vi "MS SQL_InRFID_STN30B.vi"(6 "RFID":string, 7 "OP30B_006_CIRCLIP_MEAS":T1, 8 "error in (no error)":errorcluster, 11 "Ref in":T2={"MS SQL Connection"=refnum, "UDL File"=path "", "Time"="", "DCODE"="", "WIP+1"=0, "MC No?"=0, "POKAYOKE?"=FALSE, "Expected Result"="", "Result [Status]"="", "Clock"=0.0, "RFID"="", "WIP Queue"=refnum, "TS Parameter"={"ProfitCenterCode"="", "LineCode"="", "WorkOrderNumber"="", "Model"="", "Model_with_Prefix"="", "VendorCode"="", "SetParameterDateCode"="", "PokaYoke"=0, "Target"=1, "Live_DateCode"="", "CustomerPartNumber"="", "Hand"="", "Ent_Stamp"=timestamp(0 s since 1904-01-01), "STS_CD"=0.0}, "Data_Queue"=[], "RFID Serial No."=""} {"TS Parameter"."Target" min=1 max=100000; "TS Parameter"."PokaYoke" min=0 max=1}) -> (0 "error out":errorcluster, 1 "Message":picture, 3 "Ref Out":T2={"MS SQL Connection"=refnum, "UDL File"=path "", "Time"="", "DCODE"="", "WIP+1"=0, "MC No?"=0, "POKAYOKE?"=FALSE, "Expected Result"="", "Result [Status]"="", "Clock"=0.0, "RFID"="", "WIP Queue"=refnum, "TS Parameter"={"ProfitCenterCode"="", "LineCode"="", "WorkOrderNumber"="", "Model"="", "Model_with_Prefix"="", "VendorCode"="", "SetParameterDateCode"="", "PokaYoke"=0, "Target"=1, "Live_DateCode"="", "CustomerPartNumber"="", "Hand"="", "Ent_Stamp"=timestamp(0 s since 1904-01-01), "STS_CD"=0.0}, "Data_Queue"=[], "RFID Serial No."=""} {"TS Parameter"."Target" min=1 max=100000; "TS Parameter"."PokaYoke" min=0 max=1})   [LabVIEW 2020]
uses:
  Controls/TD SQL.ctl
  <vilib>/addons/database/Connection.llb/Conn ObjectReference.ctl
  Controls/WIP_State.ctl
  Controls/TS_Parameter.ctl
  Controls/OP30B_DataCluster.ctl
  <vilib>/addons/database/NI_Database_API.lvlib
panel:
  out "OP30B VISION STATUS":i32
  out "resulting string":string
  # "OP60"
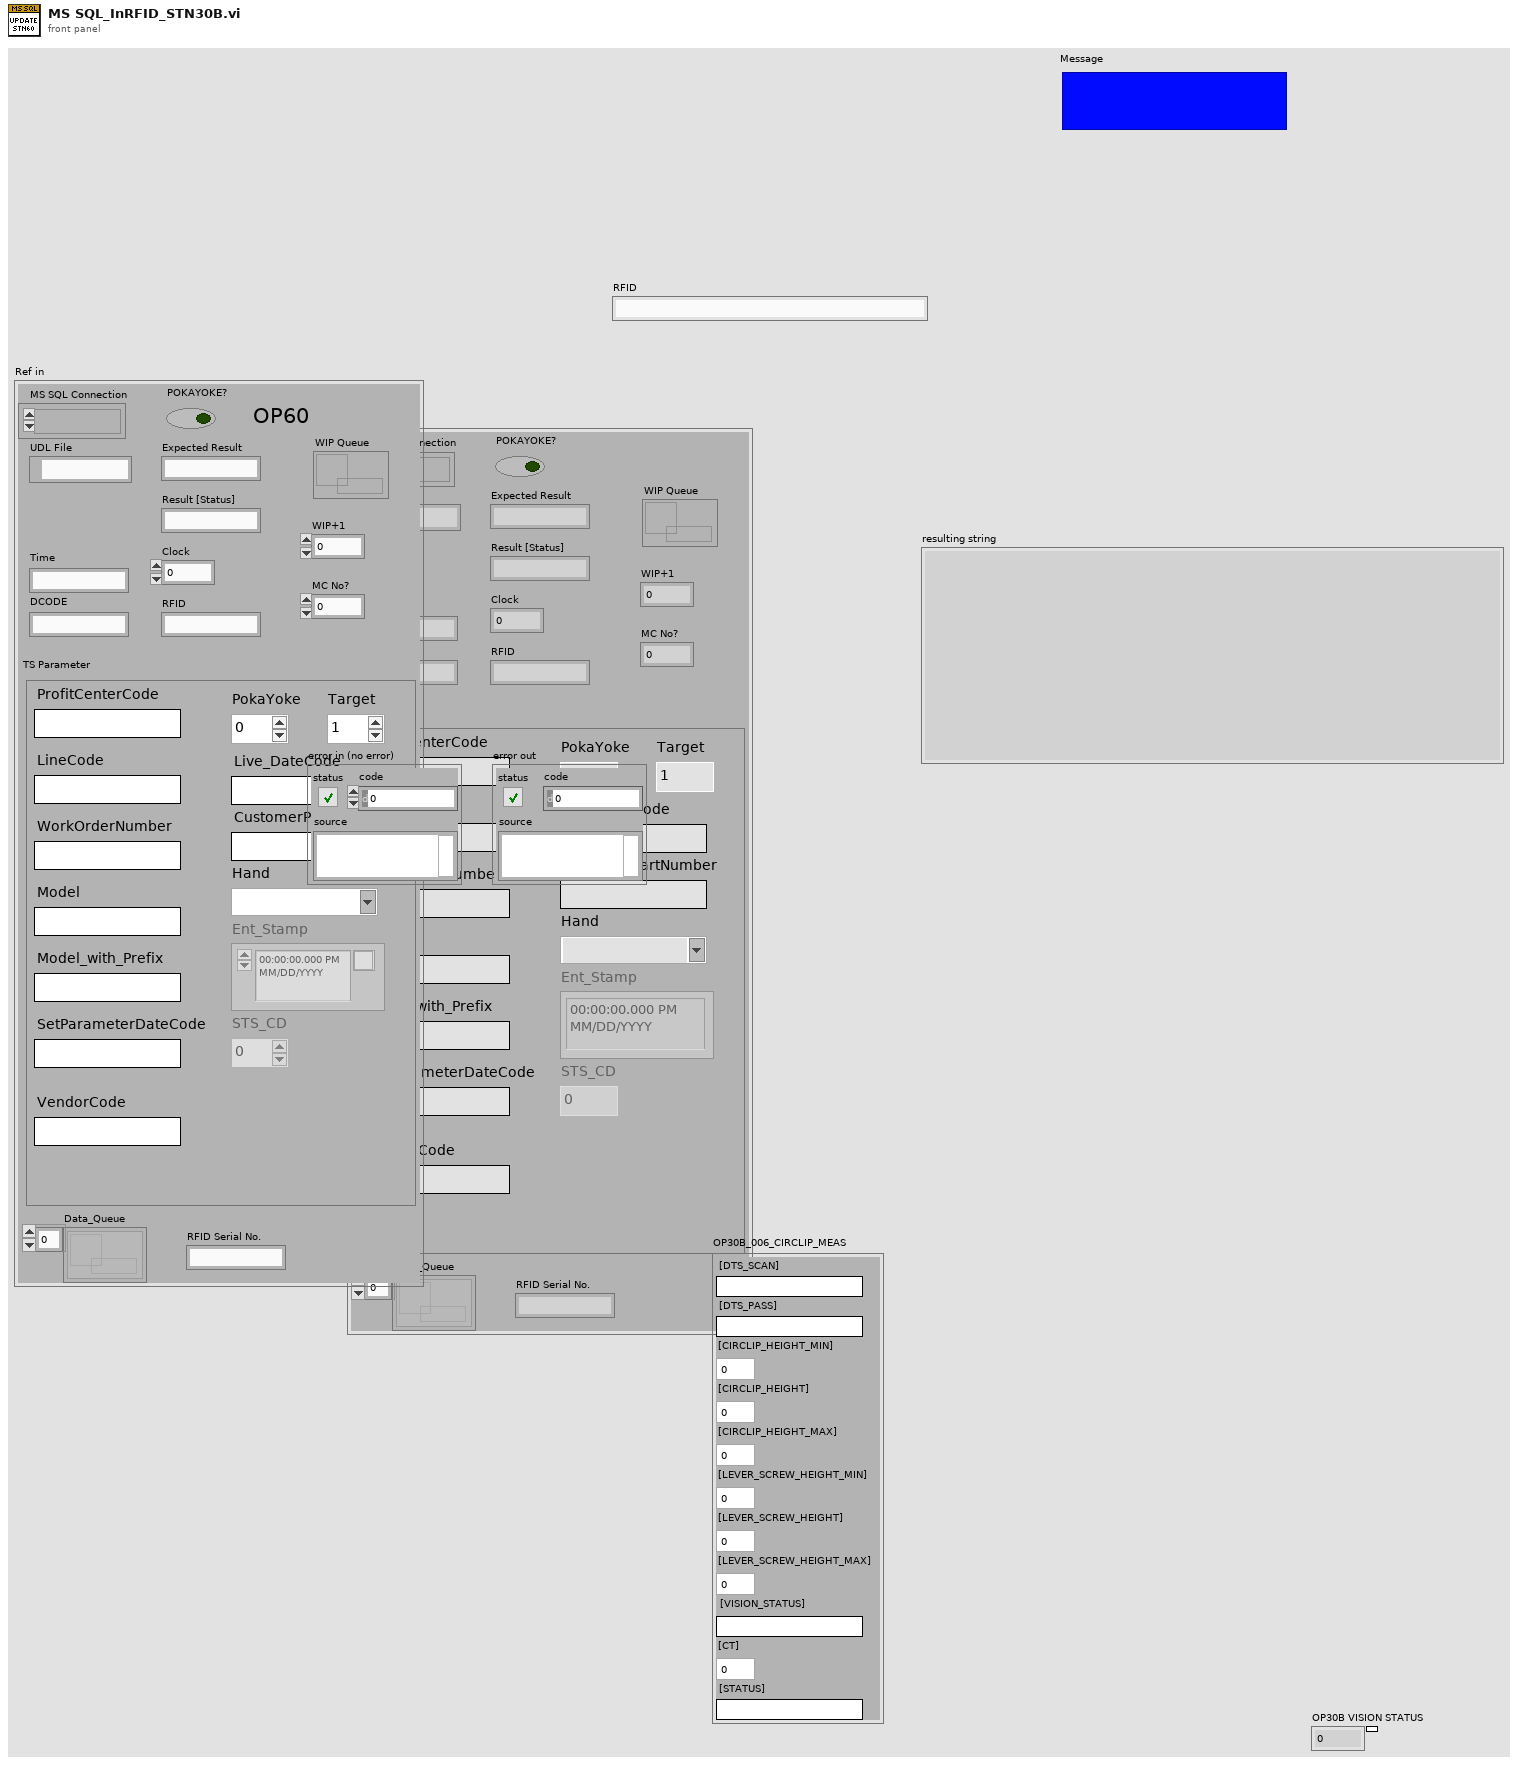
[diagram p1: front panel]
types:
  T1 = typedef "OP30B_DataCluster.ctl" = cluster{"[DTS_SCAN]":string, "[DTS_PASS]":string, "[CIRCLIP_HEIGHT_MIN]":dbl, "[CIRCLIP_HEIGHT]":dbl, "[CIRCLIP_HEIGHT_MAX]":dbl, "[LEVER_SCREW_HEIGHT_MIN]":dbl, "[LEVER_SCREW_HEIGHT]":dbl, "[LEVER_SCREW_HEIGHT_MAX]":dbl, "[VISION_STATUS]":string, "[CT]":dbl, "[STATUS]":string}
  T2 = typedef "TD SQL.ctl" = cluster{"MS SQL Connection":T3, "UDL File":path, "Time":string, "DCODE":string, "WIP+1":i64, "MC No?":i32, "POKAYOKE?":bool, "Expected Result":string, "Result [Status]":string, "Clock":dbl, "RFID":string, "WIP Queue":refnum<queue>, "TS Parameter":T4, "Data_Queue":refnum<queue>[], "RFID Serial No.":string}
  T3 = typedef "NI_Database_API.lvlib/Conn ObjectReference.ctl" = refnum<k1>
  T4 = typedef "TS_Parameter.ctl" = cluster{"ProfitCenterCode":string, "LineCode":string, "WorkOrderNumber":string, "Model":string, "Model_with_Prefix":string, "VendorCode":string, "SetParameterDateCode":string, "PokaYoke":i32, "Target":i32, "Live_DateCode":string, "CustomerPartNumber":string, "Hand":string, "Ent_Stamp":timestamp, "STS_CD":dbl}
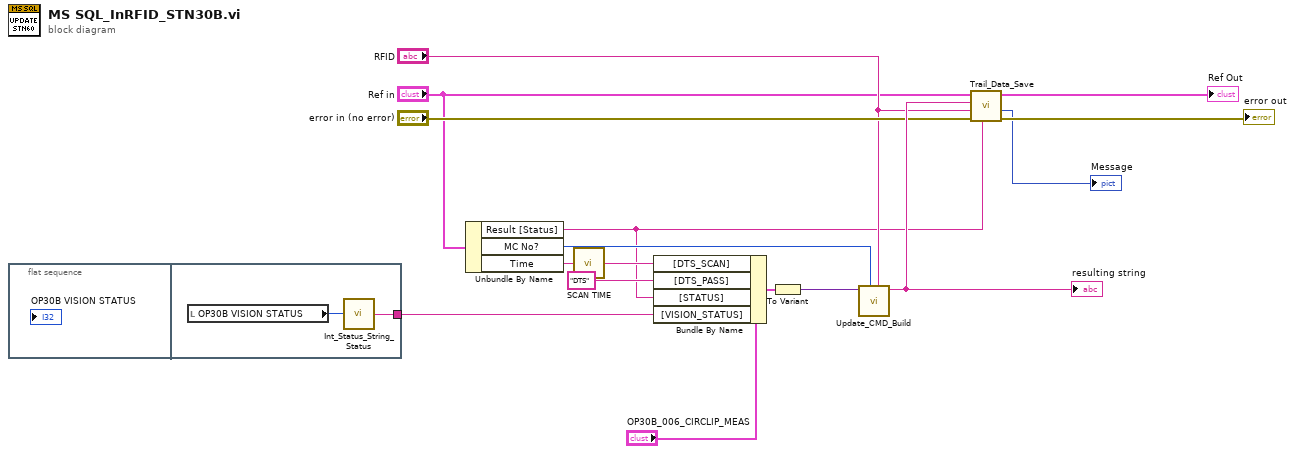
[diagram p0: block diagram]
diagram:
  n1 = flat-sequence {
    tunnel: [w17] -> w3
    frame #0 {
    }
    frame #1 {
      n2 = local read "OP30B VISION STATUS"() -> (w18:i32)
      n3 = call "Int_Status_String_Status.vi"("[STATUS]"=w18) -> ("STATUS"=w17:string)
    }
  }
  n4 = Unbundle By Name("Ref in") -> ("Result [Status]"=w1:string, "MC No?"=w2:i32, "Time"=w6:string)
  n5 = call "SCAN TIME.vi"("Time in"=w6) -> ("Time out"=w13:string)
  n6 = Bundle By Name(cluster="OP30B_006_CIRCLIP_MEAS", "[DTS_SCAN]"=w13, "[DTS_PASS]"="DTS", "[STATUS]"=w1, "[VISION_STATUS]"=w3) -> (w16:T1)
  n7 = To Variant(anything=w16) -> (Variant=w14:variant)
  n8 = call "Update_CMD_Build.vi"("RFID"="RFID", "Machine No"=w2, "Variant"=w14) -> ("Update Query"=w11:string)  [unwired: 5 in, 1 out]
  "resulting string" <- w11
  n9 = call "Trail_Data_Save.vi"("Status"=w1, "error in (no error)"="error in (no error)", "RFID"="RFID", "Query"=w11, "Ref in"="Ref in") -> ("error out"=→"error out":errorcluster, "Message"=→"Message":picture, "Ref Out"=→"Ref Out":T2)  [unwired: 1 in, 1 out]
